vi "OP400ZP_OCVmin.vi"() -> ()   [LabVIEW 2020]
panel:
  out "OCVmin":dbl
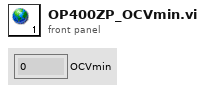
[diagram p1: front panel]
diagram:
